vi "Interprete message.vi"(8 "error in (no error)":errorcluster, 11 "TCS_ACS in":refnum<class "TCS.lvclass">) -> (0 "error out":errorcluster, 3 "TCS_ACS out":refnum<class "TCS.lvclass">)   [LabVIEW 2018, in "TCS.lvclass"]
uses:
  TCS.lvclass
  TCS.lvclass/TCS.ctl
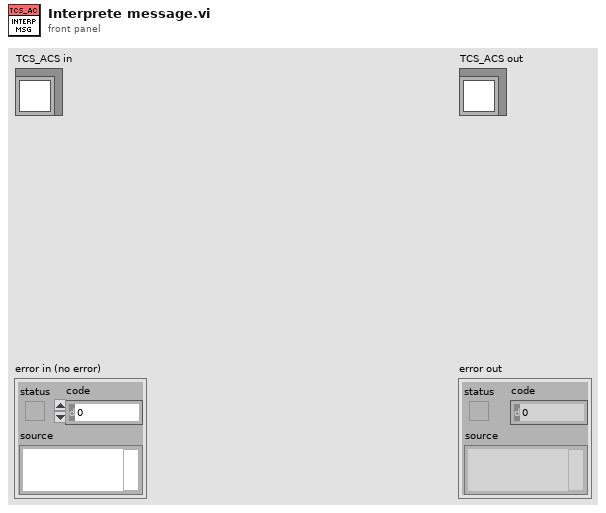
[diagram p1: front panel]
types:
  T1 = cluster{"OBJ":string, "RA":string, "DEC":string, "EPOCH":dbl, "AIRMASS":dbl, "JD":dbl, "SD":string, "HA":string, "TCSDATE":string, "FOCUS":string, "WS_DEFAULT":string, "TEMP":string, "BAR":string, "HUM":string, "FILTER":string, "CTRLINTE":string}
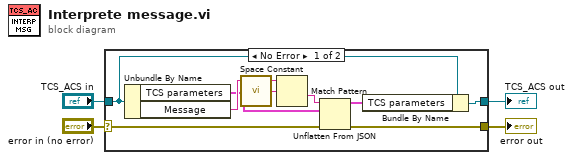
[diagram p0: block diagram]
diagram:
  n1 = case shown="No Error" "error in (no error)" {
    selector: "error in (no error)" -> [w9 w15]
    tunnel: [w8 w15] -> w3
    tunnel: [w10 w14] -> w1
    tunnel: "TCS_ACS in" -> [w11 w14]
    frame No Error {
      n2 = Unbundle By Name(w11) -> ("TCS parameters"=w6:T1, "Message"=w13:string)
      n3 = call <vilib>:"Space Constant.vi"() -> ("String"=w12:string)
      n4 = Match Pattern(string=w13, regular expression=w12) -> (after substring=w7:string)  [unwired: 1 in, 3 out]
      n5 = Unflatten From JSON(JSON string=w7, type and defaults=w6, error in (no error)=w9) -> (value=w5:T1, error out=w8:errorcluster)  [unwired: 4 in]
      n6 = Bundle By Name(cluster=w11, "TCS parameters"=w5) -> (w10:refnum<class "TCS.lvclass">)
    }
    frame Error {
    }
  }
  "error out" <- w3
  "TCS_ACS out" <- w1
